vi "ws_set_use.vi"(3 "user":string, 4 "in_use":bool, 5 "target_name":string) -> (0 "Error_info":string, 1 "Error?":bool, 2 "success":bool)   [LabVIEW 2011]
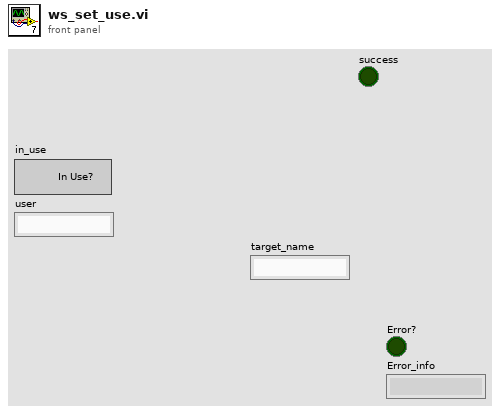
[diagram p1: front panel]
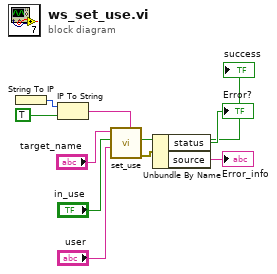
[diagram p0: block diagram]
diagram:
  n1 = String To IP() -> (0:w10:u32)  [unwired: 1 in]
  n2 = IP To String(1:TRUE ("dot notation? (F)"), 2:w10) -> (0:w5:string)
  n3 = call "set_use.vi"("Remote Server Address"=w5, "User"="user", "In Use?"="in_use", "Target Name"="target_name") -> ("error out"=w6:errorcluster, "success"=→"success":bool)  [unwired: 5 in]
  n4 = Unbundle By Name(w6) -> ("status"=→"Error?":bool, "source"=→"Error_info":string)
